vi "screen for automatic display mode.vi"() -> ()   [LabVIEW 2022 SP3]
uses:
  procedurre control.ctl
panel:
  out "procedurre array":cluster{"Job Name Cluster":T1}[](array[cluster]) {"Job Name Cluster"."?" format="%#.6f"; "Job Name Cluster"."?" format="%#.6f"; "Job Name Cluster"."?" format="%#.6f"; "Job Name Cluster"."?" format="%#.6f"}
  in  "back":bool
  in  "Xaxis progress":dbl(slide) scale=0.0..10.0
  in  "yaxis progress":dbl(slide) scale=0.0..10.0
  out "total procedure":dbl format="%#.6f"
  out "current procedure":dbl format="%#.6f"
  out "outoff":dbl format="%#.6f"
  out "current no":dbl format="%#.6f"
  out "procedure status":bool
  out "Name of procedure":string="Job name Line 1 Line 2"
  out "started time":timestamp format="%<%d %b %Y | %H:%M>T"
  out "Remaining time":timestamp format="%<%-%Hh %Mm %Ss>T"
  out "Y axis":picture
  out "x axis":picture
  # "Procedures completed"
  # "/"
  # "STEPS"
  # "CYCLES"
  # "/"
  # "/"
  # "/"
  # "JOB STARTED ON"
  # "Remaining"
  # "Y Axis"
  # "X Axis"
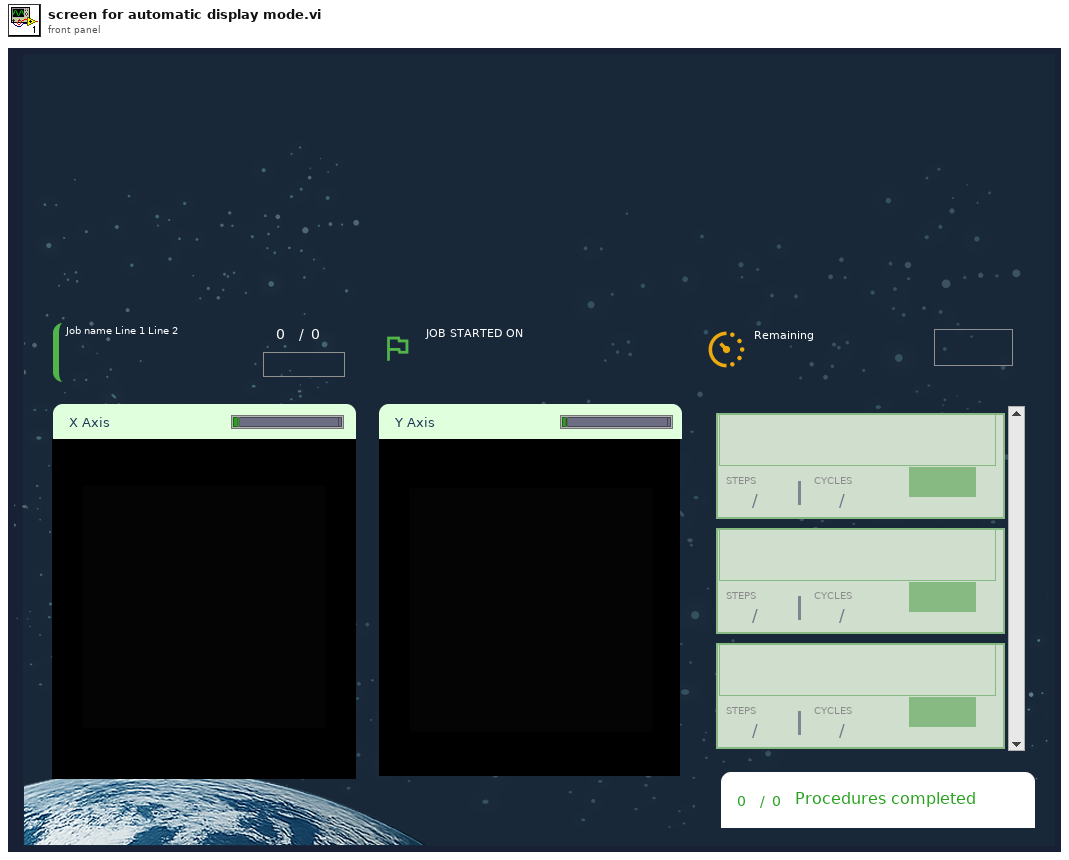
[diagram p1: front panel]
types:
  T1 = typedef "procedurre control.ctl" = cluster{string, dbl, dbl, dbl, dbl, "Enum":enum16{"Done", "Active", "Next"}}
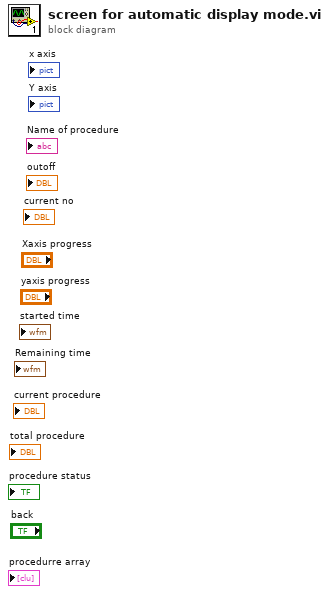
[diagram p0: block diagram]
diagram:
